vi "Create.vi"(8 "Error In":errorcluster, 11 "Reader":refnum<class "Abstract.lvclass">) -> (0 "Error Out":errorcluster, 3 "Parser":refnum<class "Lexer.lvclass">)   [LabVIEW 2018, in "Toolkit.lvlib" / "Lexer.lvclass"]
uses:
  Lexer.lvclass
  Readers/Abstract/Abstract.lvclass
  Lexer.lvclass/Lexer.ctl
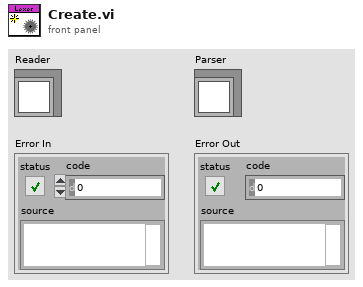
[diagram p1: front panel]
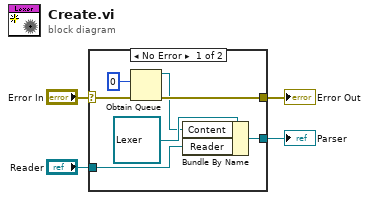
[diagram p0: block diagram]
diagram:
  n1 = case shown="No Error" "Error In" {
    selector: "Error In" -> [w8 w12]
    tunnel: [w7 w12] -> w3
    tunnel: [w9 _] -> w2
    tunnel: "Reader" -> [w10 _]
    frame No Error {
      n2 = Obtain Queue(element data type=u8 0, error in (no error)=w8) -> (queue out=w5:refnum<queue>, error out=w7:errorcluster)  [unwired: 3 in, 1 out]
      n3 = Bundle By Name(cluster=refnum<class "Lexer.lvclass"> refnum ("Mustache.lvlib:Parser.lvclass"), "Content"=w5, "Reader"=w10) -> (w9:refnum<class "Lexer.lvclass">)
    }
    frame Error {
    }
  }
  "Error Out" <- w3
  "Parser" <- w2
